vi "传感器映射 彩色云图.vi"(1 "液罐":dbl(slide) scale=0.0..10.0) -> (0 "三维图片":refnum<vi>(3d-picture))   [LabVIEW 2019]
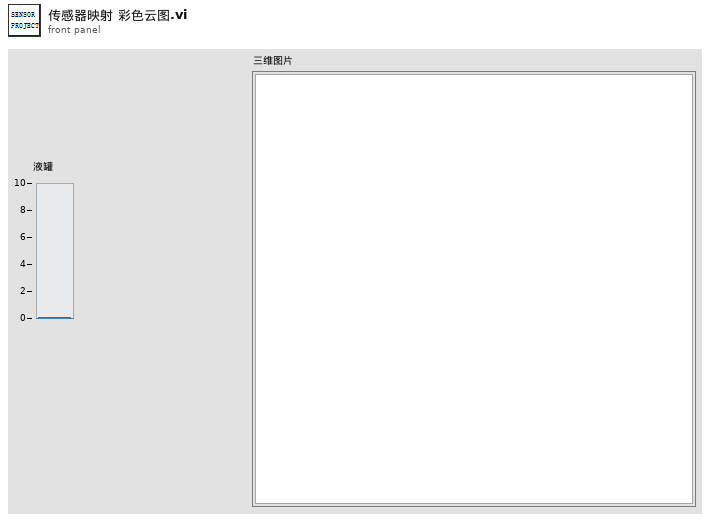
[diagram p1: front panel]
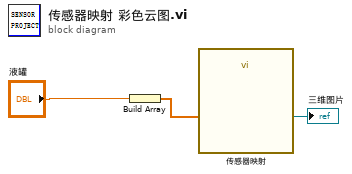
[diagram p0: block diagram]
diagram:
  n1 = Build Array("液罐") -> (w2:dbl[])
  n2 = call "传感器映射"("Sensor Values"=w2) -> ("Scene Ref Out"=→"三维图片":refnum<vi>)  [unwired: 9 in, 1 out]
